vi "Stop Core.vi"(10 "final error code":i32, 11 "CS++PVProxy in":refnum<class "CS++PVProxy.lvclass">) -> (3 "CS++PVProxy out":refnum<class "CS++PVProxy.lvclass">)   [LabVIEW 2016, in "CS++PVProxy.lvlib" / "CS++PVProxy.lvclass"]
doc: "(<B>Filename</B>: Actor Framework.lvlib:Actor.lvclass:Stop Core.vi)\n\nDefines what the actor does before it stops. Use the <B>final error code</B> input to determine whether the actor shut down in response to an error.\n\nBy default, this method does nothing. A descendant class may override it to define behavior, such as shutting down any processes the actor initiated in its override of the Actor Core method."
uses:
  CS++PVProxy.lvclass
  CS++PVProxy.lvclass/CS++PVProxy.ctl
  CS++BaseActor/CS++BaseActor.lvclass
  Classes/CS++ProcessVariables/PVConnection/PVConnection.lvclass
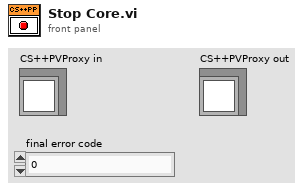
[diagram p1: front panel]
types:
  T1 = cluster{"Name":string, "Polling-String":string, "CS++PVUpdate Msg":refnum<class "CS++PVUpdate Msg.lvclass">, "PVConnection":refnum<class "PVConnection.lvclass">}[]
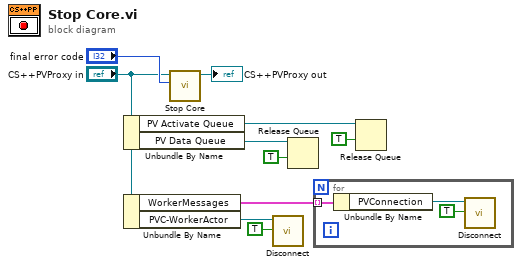
[diagram p0: block diagram]
diagram:
  n1 = Unbundle By Name("CS++PVProxy in") -> ("PV Activate Queue"=w8:refnum<queue>, "PV Data Queue"=w7:refnum<queue>)
  n2 = Unbundle By Name("CS++PVProxy in") -> ("WorkerMessages"=w3:T1, "PVC-WorkerActor"=w1:refnum<class "PVConnection.lvclass">)
  n3 = call-parent "Stop Core.vi"("final error code"="final error code", "CS++BaseActor in"="CS++PVProxy in") -> ("CS++BaseActor out"=→"CS++PVProxy out":refnum<class "CS++PVProxy.lvclass">)  [unwired: 9 in]
  n4 = call "Disconnect.vi"("Force (T)"=TRUE, "PVConnection in"=w1) -> ()  [unwired: 8 in, 2 out]
  n5 = Release Queue(queue=w7, force destroy? (F)=TRUE) -> ()  [unwired: 1 in, 3 out]
  n6 = for {
    tunnel: w3 -> [w13] mode=indexing
    n7 = Unbundle By Name(w13) -> ("PVConnection"=w11:refnum<class "PVConnection.lvclass">)
    n8 = call "Disconnect.vi"("Force (T)"=TRUE, "PVConnection in"=w11) -> ()  [unwired: 8 in, 2 out]
  }
  n9 = Release Queue(queue=w8, force destroy? (F)=TRUE) -> ()  [unwired: 1 in, 3 out]
